vi "sub_GNSS-Serial.vi"(8 "error in":errorcluster) -> (0 "error out":errorcluster)   [LabVIEW 2019]
uses:
  Ctrl/cmd_RW.ctl
  Ctrl/cmd_common.ctl
  Ctrl/cmd_ini-RW.ctl
  Ctrl/cmd_ini-add-read.ctl
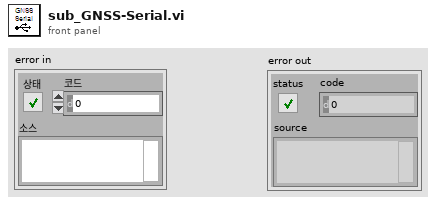
[diagram p1: front panel]
types:
  T1 = typedef "cmd_ini-RW.ctl" = enum16{"ini", "read", "write"}
  T2 = typedef "cmd_common.ctl" = enum16{"read", "write"}
  T3 = typedef "cmd_RW.ctl" = enum16{"read", "write"}
  T4 = typedef "cmd_ini-add-read.ctl" = enum16{"ini", "add", "read"}
  T5 = cluster{"GxGGA":string, "GxGSV":string, "GNRMC":string, "GxTXT":string, "GxGSA":string, "GxGLL":string}
  T6 = typedef "GNSS-Ntrip config.ctl" = cluster{"Ntrip accounts DB":T7[], "Mount points":u16, "Ref r size":dbl, "TMarr limit":i32, "Sel NMEA type":enum16{"$GPGSV", "$GLGSV", "$GPGGA", "$GAGSV", "$GBGSV", "$GNGLL", "$GNGGA", "$GNGSA", "$GNRMC", "$GNVTG"}, "Local Time offset":u32, "GNSS Serial delay":u32, "Send Serial delay":u32, "Send Serial config":cluster{"NMEA out port":refnum<visa-resource-name>, "baud rate":u32}, "Mount point arr":string[], "Ntrip account DB index":u32}
  T7 = typedef "Ntrip_Account_db.ctl" = cluster{"address":string, "port ":u16, "id":string, "pwd":string, "ref pt":string}
  T8 = enum16{"$GPGSV", "$GLGSV", "$GPGGA", "$GAGSV", "$GBGSV", "$GNGLL", "$GNGGA", "$GNGSA", "$GNRMC", "$GNVTG"}
  T9 = typedef "GNSS-Ntrip process val.ctl" = cluster{"GNSS time":string, "Ntrip conn":bool, "NMEA val":bool, "ycenter_TM":dbl, "xcenter_TM":dbl, "TM ref circles":cluster{"Y(E)":dbl, "X(N)":dbl}[], "RTCM recv-str":string, "GNSS Serail buff N":u32, "Sel NMEA type":enum16{"$GPGSV", "$GLGSV", "$GPGGA", "$GAGSV", "$GBGSV", "$GNGLL", "$GNGGA", "$GNGSA", "$GNRMC", "$GNVTG"}, "RTCM recv_sourcetable":string, "NMEA cluster":cluster{"GxGGA":string, "GxGSV":string, "GNRMC":string, "GxTXT":string, "GxGSA":string, "GxGLL":string}, "Sel NMEA str":string, "NMEA recv-str":string}
  T10 = cluster{"Ntrip tcp":bool, "GNSS serial":bool, "RTCM serial":bool, "Send serial":bool}
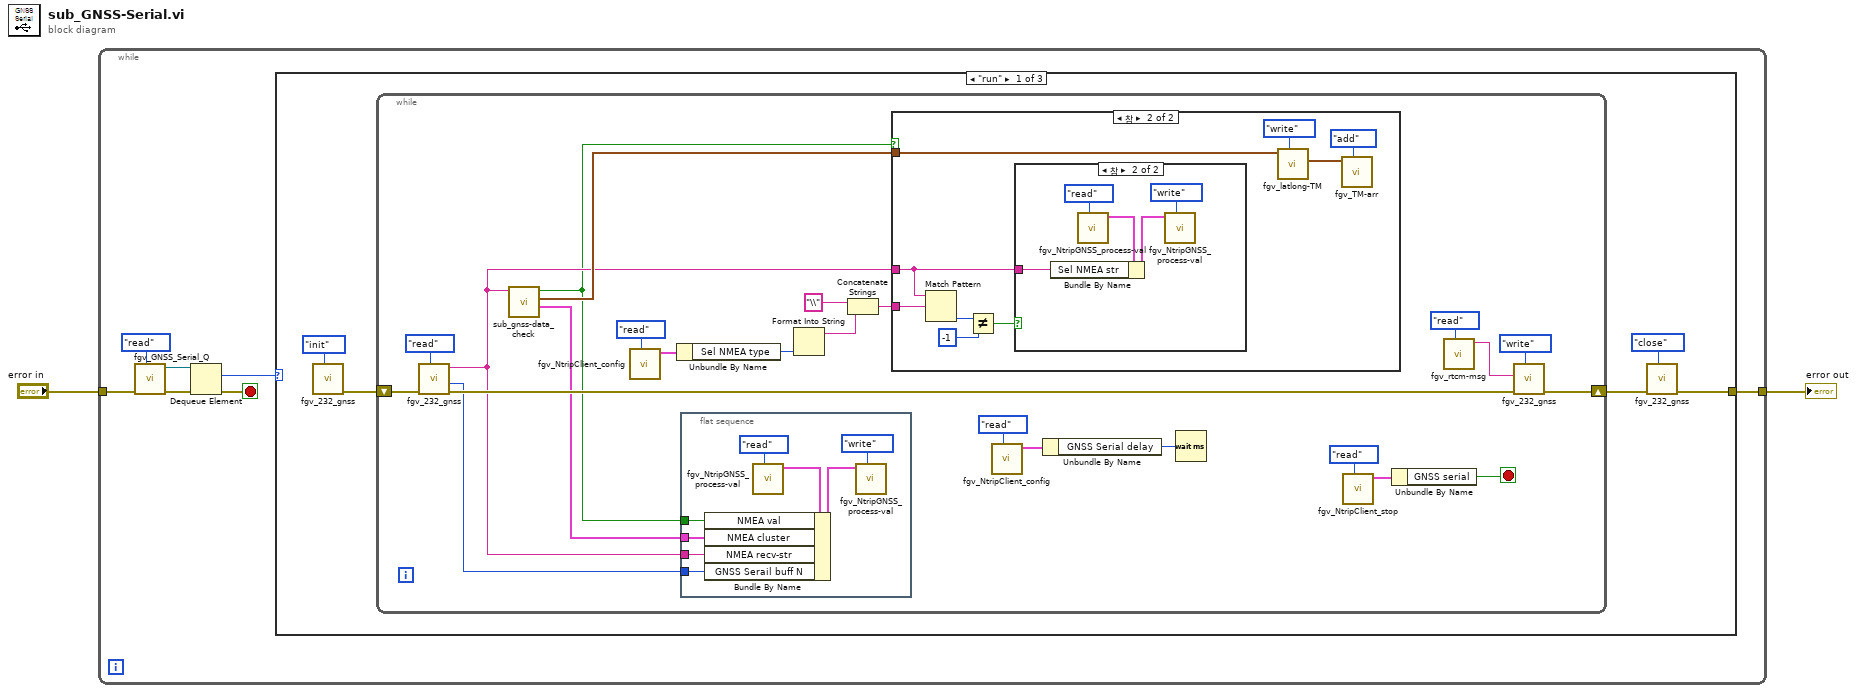
[diagram p0: block diagram]
diagram:
  n1 = while {
    tunnel: "error in" -> [w6]
    tunnel: [w3] -> w1
    stop <- w4 stop-if-true
    n2 = call "fgv_GNSS_Serial_Q.vi"("cmd"=enum16{"create", "write", "read", "close"}."read", "error in"=w6) -> ("error out"=w5:errorcluster, "queue out"=w9:refnum<queue>)  [unwired: 8 in]
    n3 = Dequeue Element(queue=w9, error in (no error)=w5) -> (element=w7:enum16{"run", "check", "stop"}, error out=w4:errorcluster)  [unwired: 1 in, 2 out]
    n4 = case shown="\"run\"" w7 {
      tunnel: [w10 _ _] -> w3
      frame "run" {
        n5 = call "fgv_232_gnss.vi"("cmd"=enum16{"init", "read", "write", "close"}."init") -> ("error out"=w13:errorcluster)  [unwired: 8 in, 2 out]
        n6 = while {
          shift-right: [w28] -> w11
          shift-left: w13 -> [w37]
          stop <- w15 stop-if-true
          n7 = call "fgv_232_gnss.vi"("cmd"=enum16{"init", "read", "write", "close"}."read", "error in"=w37) -> ("error out"=w31:errorcluster, "byte n"=w27:u32, "read_buffer"=w25:string)  [unwired: 7 in]
          n8 = call "sub_gnss-data_check.vi"("gnss str"=w25) -> ("NMEA cluster"=w24:T5, "LatLong"=w36:cluster{dbl, dbl}, "val"=w18:bool)  [unwired: 7 in, 1 out]
          n9 = call "fgv_NtripClient_config.vi"("cmd"=cmd_common."read") -> ("config val out"=w20:T6)  [unwired: 10 in]
          n10 = Unbundle By Name(w20) -> ("Sel NMEA type"=w19:T8)
          n11 = flat-sequence {
            tunnel: w27 -> [w42]
            tunnel: w25 -> [w41]
            tunnel: w24 -> [w40]
            tunnel: w18 -> [w39]
            frame #0 {
              n12 = call "fgv_NtripGNSS_process-val.vi"("cmd"=cmd_ini-RW."read") -> ("process val out"=w46:T9)  [unwired: 10 in]
              n13 = Bundle By Name(cluster=w46, "NMEA val"=w39, "NMEA cluster"=w40, "NMEA recv-str"=w41, "GNSS Serail buff N"=w42) -> (w45:T9)
              n14 = call "fgv_NtripGNSS_process-val.vi"("cmd"=cmd_ini-RW."write", "process val"=w45) -> ()  [unwired: 9 in, 1 out]
            }
          }
          n15 = Format Into String(w19) -> (resulting string=w35:string)  [unwired: 3 in, 1 out]
          n16 = Concatenate Strings("\\" ("string"), w35) -> (w33:string)
          n17 = case shown="참" w18 {
            tunnel: w25 -> [_ w49]
            tunnel: w36 -> [_ w54]
            tunnel: w33 -> [_ w53]
            frame False {
            }
            frame True {
              n18 = Match Pattern(string=w49, regular expression=w53) -> (offset past match=w52:i32)  [unwired: 1 in, 3 out]
              n19 = Not Equal?(x=w52, y=-1) -> (x != y?=w50:bool)
              n20 = case shown="참" w50 {
                tunnel: w49 -> [_ w56]
                frame False {
                }
                frame True {
                  n21 = call "fgv_NtripGNSS_process-val.vi"("cmd"=cmd_ini-RW."read") -> ("process val out"=w60:T9)  [unwired: 10 in]
                  n22 = Bundle By Name(cluster=w60, "Sel NMEA str"=w56) -> (w59:T9)
                  n23 = call "fgv_NtripGNSS_process-val.vi"("cmd"=cmd_ini-RW."write", "process val"=w59) -> ()  [unwired: 9 in, 1 out]
                }
              }
              n24 = call "fgv_latlong-TM.vi"("cmd"=enum16{"write", "read"}."write", "latlong"=w54) -> ("tm out"=w47:cluster{"YE":dbl, "XN":dbl})  [unwired: 8 in, 1 out]
              n25 = call "fgv_TM-arr.vi"("cmd"=cmd_ini-add-read."add", "TM"=w47) -> ()  [unwired: 9 in, 1 out]
            }
          }
          n26 = call "fgv_NtripClient_config.vi"("cmd"=cmd_common."read") -> ("config val out"=w22:T6)  [unwired: 10 in]
          n27 = Unbundle By Name(w22) -> ("GNSS Serial delay"=w26:u32)
          n28 = Wait (ms)(milliseconds to wait=w26) -> ()  [unwired: 1 out]
          n29 = call "fgv_NtripClient_stop.vi"("cmd"=cmd_ini-RW."read") -> ("local stops out"=w17:T10)  [unwired: 10 in]
          n30 = Unbundle By Name(w17) -> ("GNSS serial"=w15:bool)
          n31 = call "fgv_rtcm-msg.vi"("cmd"=cmd_RW."read") -> ("rtcm msg out"=w29:string)  [unwired: 10 in]
          n32 = call "fgv_232_gnss.vi"("cmd"=enum16{"init", "read", "write", "close"}."write", "error in"=w31, "write buff"=w29) -> ("error out"=w28:errorcluster)  [unwired: 6 in, 2 out]
        }
        n33 = call "fgv_232_gnss.vi"("cmd"=enum16{"init", "read", "write", "close"}."close", "error in"=w11) -> ("error out"=w10:errorcluster)  [unwired: 7 in, 2 out]
      }
      frame "check" {
      }
      frame "stop", Default {
      }
    }
  }
  "error out" <- w1
